vi "Unregister IRQ.vi"(8 "error in (no error)":errorcluster, 11 "IRQ Number":u8) -> (0 "error out":errorcluster)   [LabVIEW 2021, in "IO IRQ.lvlib"]
doc: "Unregisters analog and digital input interrupts. After you unregister an interrupt, LabVIEW stops registering the interrupt."
uses:
  <vilib>/myRIO/Instrument Drivers/IRQ/IO IRQ/IO IRQ.lvlib
  <vilib>/myRIO/Common/Instrument Driver Framework/Utilities/typedefs/FPGA Ref Manager Action Enum.ctl
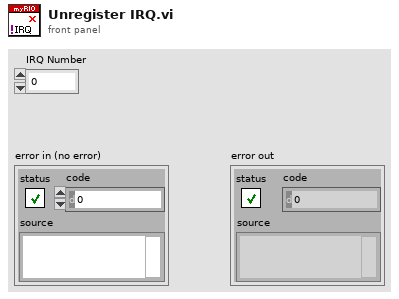
[diagram p1: front panel]
types:
  T1 = typedef "FPGA Ref Manager Action Enum.ctl" = enum16{"Get", "Set", "Reset"}
  T2 = typedef "Generic FPGA Reference.ctl" = refnum<k20>
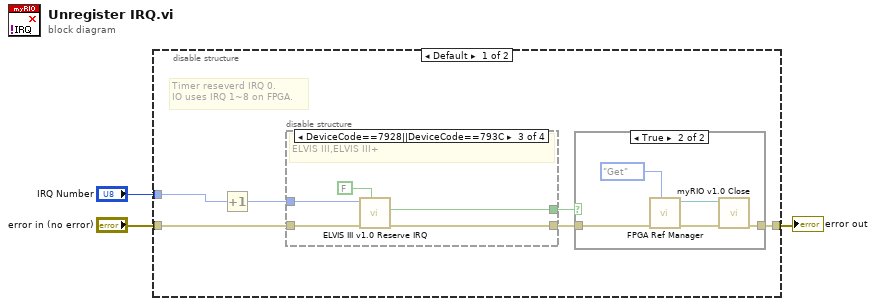
[diagram p0: block diagram]
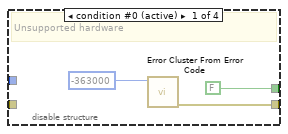
[diagram p2: hidden frame]
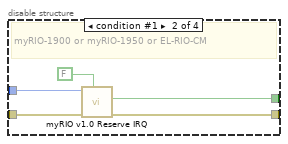
[diagram p3: hidden frame]
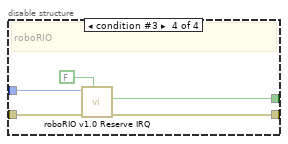
[diagram p4: hidden frame]
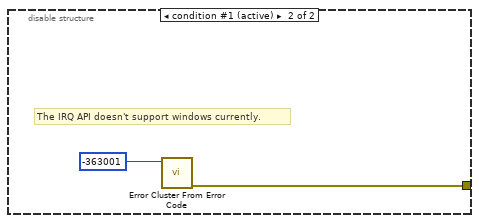
[diagram p6: hidden frame]
diagram:
  n1 = disable-structure shown="Default" {
    disable-tunnel: [w9 w34] -> w3
    disable-tunnel: "IRQ Number" -> [w8 _]
    disable-tunnel: "error in (no error)" -> [w5 _]
    frame condition #0 {
      # "Timer reseverd IRQ 0.\nIO uses IRQ 1~8 on FPGA."
      n2 = Increment(x=w8) -> (x+1=w7:u8)
      n3 = disable-structure shown="DeviceCode==7928||DeviceCode==793C" {
        disable-tunnel: w7 -> [_ w17 w21 w27]
        disable-tunnel: [FALSE ("Succeed?") w16 w19 w26] -> w6
        disable-tunnel: w5 -> [_ w15 w20 w25]
        disable-tunnel: [w11 w14 w18 w24] -> w4
        frame condition #0 (active) {
          # "Unsupported hardware"
          n4 = call <vilib>:"Error Cluster From Error Code.vi"("error code (0)"=-363000) -> ("error out"=w11:errorcluster)  [unwired: 8 in]
        }
        frame condition #1 {
          # "myRIO-1900 or myRIO-1950 or EL-RIO-CM"
          n5 = call <vilib>:"myRIO v1.0 Reserve IRQ.vi"("Is Reserve?"=FALSE, "error in (no error)"=w15, "IRQ Number"=w17) -> ("error out"=w14:errorcluster, "Succeed?"=w16:bool)  [unwired: 7 in]
        }
        frame condition #2 {
          # "ELVIS III,ELVIS III+"
          n6 = call <vilib>:"ELVIS III v1.0 Reserve IRQ.vi"("Is Reserve?"=FALSE, "error in (no error)"=w20, "IRQ Number"=w21) -> ("error out"=w18:errorcluster, "Succeed?"=w19:bool)  [unwired: 7 in]
        }
        frame condition #3 {
          # "roboRIO"
          n7 = call <vilib>:"roboRIO v1.0 Reserve IRQ.vi"("Is Reserve?"=FALSE, "error in (no error)"=w25, "IRQ Number"=w27) -> ("error out"=w24:errorcluster, "Succeed?"=w26:bool)  [unwired: 7 in]
        }
      }
      n8 = case shown="True" w6 {
        tunnel: w4 -> [w28 w30]
        tunnel: [w28 w29] -> w9
        frame False {
        }
        frame True {
          n9 = call <vilib>:"FPGA Ref Manager.vi"("Action"=FPGA_Ref_Manager_Action_Enum."Get", "error in (no error)"=w30) -> ("error out"=w31:errorcluster, "Generic FPGA Reference out"=w32:T2)  [unwired: 7 in]
          n10 = call <vilib>:"myRIO v1.0 Close.vi"("error in (no error)"=w31, "myRIO FPGA Ref In"=w32) -> ("error out"=w29:errorcluster)  [unwired: 9 in]
        }
      }
    }
    frame condition #1 (active) {
      # "The IRQ API doesn't support windows currently."
      n11 = call <vilib>:"Error Cluster From Error Code.vi"("error code (0)"=-363001) -> ("error out"=w34:errorcluster)  [unwired: 8 in]
    }
  }
  "error out" <- w3
